vi "Get velocity.vi"(8 "error in (no error)":errorcluster, 11 "AlphaStep One in":refnum<class "AlphaStep One.lvclass">) -> (0 "error out":errorcluster, 2 "Velocity (rev/sec)":dbl, 3 "AlphaStep One out":refnum<class "AlphaStep One.lvclass">)   [LabVIEW 2015, in "AlphaStep One.lvclass"]
uses:
  AlphaStep One.lvclass
  AlphaStep One.lvclass/AlphaStep One.ctl
  Serial Device/Serial Device.lvclass
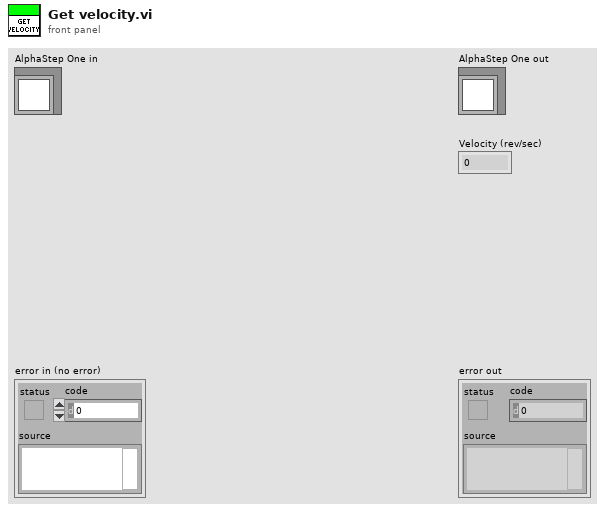
[diagram p1: front panel]
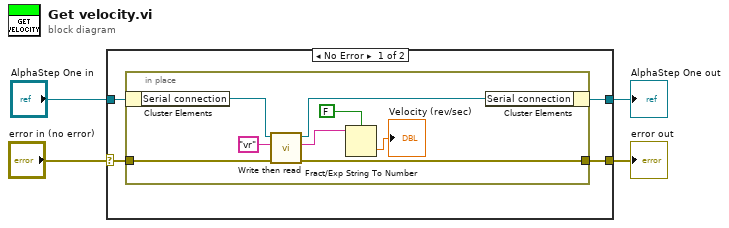
[diagram p0: block diagram]
diagram:
  n1 = case shown="No Error" "error in (no error)" {
    selector: "error in (no error)" -> [w7 w17]
    tunnel: "AlphaStep One in" -> [w8 w18]
    tunnel: [w5 w18] -> w2
    tunnel: [w6 w17] -> w1
    frame No Error {
      n2 = in-place {
        in-place-border: w7 -> [w13]
        in-place-border: [w12] -> w6
        n3 = in-place-cluster #1(w8) -> ("Serial connection"=w16:refnum<class "Serial Device.lvclass">)
        n4 = call "Write then read.vi"("error in (no error)"=w13, "TX Data"="vr", "Serial Device in"=w16) -> ("error out"=w12:errorcluster, "RX Data"=w11:string, "Serial Device out"=w15:refnum<class "Serial Device.lvclass">)  [unwired: 6 in]
        n5 = Fract/Exp String To Number(use system decimal point (T)=FALSE, string=w11) -> (number=→"Velocity (rev/sec)":dbl)  [unwired: 2 in, 1 out]
        n6 = in-place-cluster #1("Serial connection"=w15) -> (w5:refnum<class "AlphaStep One.lvclass">)
      }
    }
    frame Error {
    }
  }
  "error out" <- w1
  "AlphaStep One out" <- w2
